vi "process.vi"(8 "error in (no error)":errorcluster, 11 "LVClass in":refnum<class "LVClass.lvclass">) -> (0 "error out":errorcluster, 3 "LVClass out":refnum<class "LVClass.lvclass">)   [LabVIEW 2016, in "LVClass.lvclass"]
uses:
  LVClass.lvclass
  C:/LSST_TS/SystemSW/ct_tools/ProjectItem/ProjectItem.lvclass
  ProjectItem/ProjectItem.lvclass/ProjectItem.ctl
  Search/Search.lvclass/Search.ctl
  IProjectItemFactory/IProjectItemFactory.lvclass
  ProjectItem/ProjectItem.lvclass
  Project/Project.lvclass
  Search/Search.lvclass
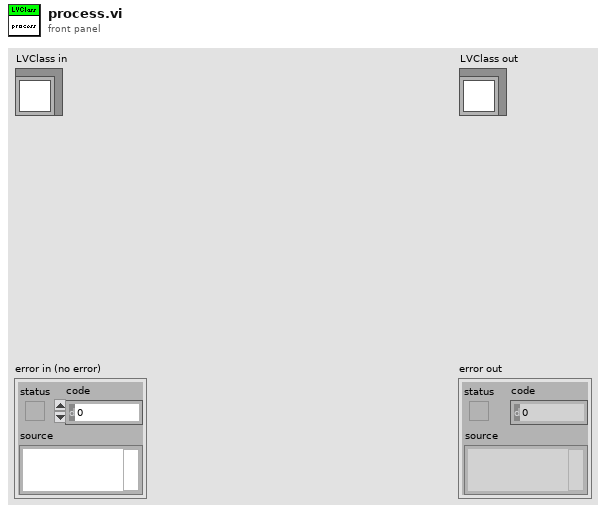
[diagram p1: front panel]
types:
  T1 = typedef "ProjectItemSelection.ctl" = enum16{"Default", "Dependencies", "Folder", "Library", "LVClass", "VI"}
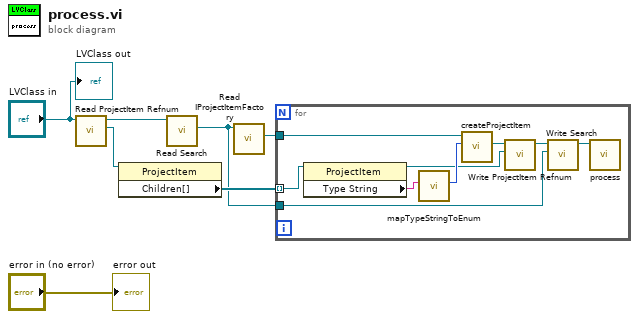
[diagram p0: block diagram]
diagram:
  n1 = call "Read ProjectItem Refnum.vi"("ProjectItem in"="LVClass in") -> ("ProjectItem Refnum"=w6:refnum<vi>, "ProjectItem out"=w3:refnum<class "LVClass.lvclass">)  [unwired: 9 in]
  n2 = property class="ProjectItem"(reference=w6) -> ("Children[]"=w5:refnum<vi>[])  [unwired: 1 in, 2 out]
  n3 = call "Read Search.vi"("ProjectItem in"=w3) -> ("Search"=w1:refnum<class "Search.lvclass">)  [unwired: 9 in, 1 out]
  n4 = call "Read IProjectItemFactory.vi"("ProjectItem in"=w1) -> ("IProjectItemFactory"=w2:refnum<class "IProjectItemFactory.lvclass">)  [unwired: 9 in, 1 out]
  n5 = for {
    tunnel: w5 -> [w16] mode=indexing
    tunnel: w2 -> [w12]
    tunnel: w1 -> [w10]
    n6 = property class="ProjectItem"(reference=w16) -> (reference out=w11:refnum<vi>, "Type String"=w15:string)  [unwired: 1 in, 1 out]
    n7 = call "mapTypeStringToEnum.vi"("Type String"=w15) -> ("ProjectItemSelection"=w14:T1)  [unwired: 8 in, 2 out]
    n8 = call-dynamic "createProjectItem.vi"("ProjectItemSelection"=w14, "IProjectItemFactory in"=w12) -> ("ProjectItem"=w13:refnum<class "ProjectItem.lvclass">)  [unwired: 7 in, 2 out]
    n9 = call "Write ProjectItem Refnum.vi"("ProjectItem Refnum"=w11, "ProjectItem in"=w13) -> ("ProjectItem out"=w9:refnum<class "ProjectItem.lvclass">)  [unwired: 9 in]
    n10 = call "Write Search.vi"("Search"=w10, "ProjectItem in"=w9) -> ("ProjectItem out"=w8:refnum<class "ProjectItem.lvclass">)  [unwired: 9 in]
    n11 = call-dynamic "process.vi"("ProjectItem in"=w8) -> ()  [unwired: 9 in, 2 out]
  }
  "error out" <- "error in (no error)"
  "LVClass out" <- "LVClass in"
